vi "Actor Core.vi"(8 "error in":errorcluster, 11 "State in":refnum<class "Operator.lvclass">) -> (0 "error out":errorcluster, 3 "Actor out":refnum<class "Actor.lvclass">)   [LabVIEW 2014, in "Operator.lvlib" / "Operator.lvclass"]
doc: "(<B>Filename</B>: Actor Framework.lvlib:Actor.lvclass:Actor Core.vi)\n\nThis override invokes Entry.vi on the initial state, prior to calling the parent Actor Core. Adding this behavior to Actor Core (instead of an override of Pre Launch Init.vi) allows the initial state to launch a nested actor as part of its entry behavior.\n\nReceives messages to the actor, reacts to them, and initiates any error handling that may shut the actor down.\n\nDescendant classes may override this VI to append parallel tasks for the actor to complete while it handles messages. Overrides use the Call Parent Method node."
uses:
  Operator.lvclass
  <vilib>/ActorFramework/Actor/Actor.lvclass
  Operator Messages/Get Operator Joystick State Msg/Get Operator Joystick State Msg.lvclass
  Operator.lvclass/Operator.ctl
  Joystick/Joystick Class/Joystick.lvclass
  Robot Actor Framework/System Actor/System Actor Class/System Actor.lvclass
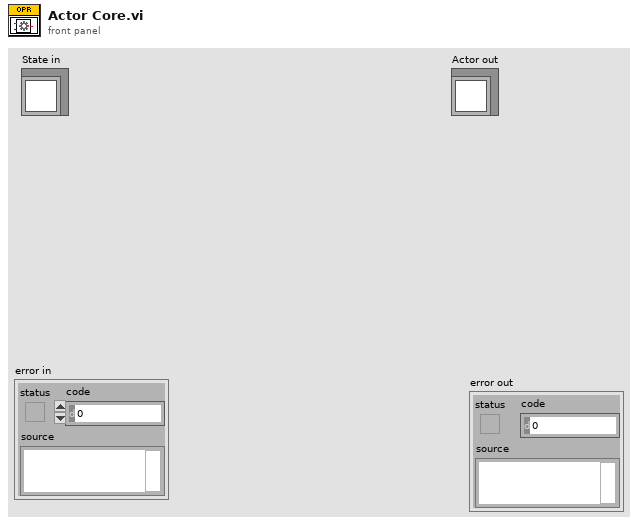
[diagram p1: front panel]
types:
  T1 = enum16{"Critical", "Error", "Warning", "Informational", "Debug"}
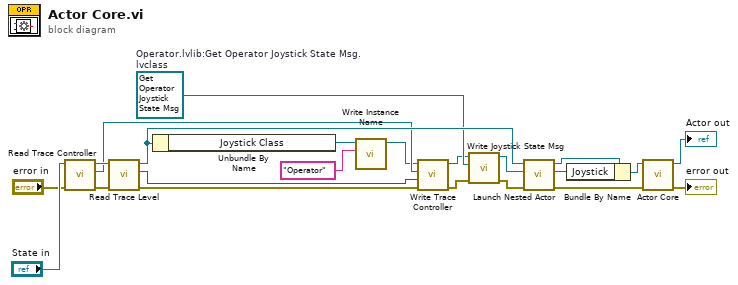
[diagram p0: block diagram]
diagram:
  w5 = refnum<class "Get Operator Joystick State Msg.lvclass"> refnum  # Operator.lvlib:Get Operator Joystick State Msg.lvclass
  n1 = call-dynamic "Read Trace Controller.vi"("error in (no error)"="error in", "System Actor in"="State in") -> ("error out"=w12:errorcluster, "Trace Controller"=w17:refnum<class "Message Enqueuer.lvclass">, "System Actor out"=w19:refnum<class "Operator.lvclass">)  [unwired: 7 in]
  n2 = call-dynamic "Read Trace Level.vi"("error in (no error)"=w12, "System Actor in"=w19) -> ("error out"=w11:errorcluster, "Trace Level"=w4:T1, "System Actor out"=w18:refnum<class "Operator.lvclass">)  [unwired: 7 in]
  n3 = Unbundle By Name(w18) -> ("Joystick Class"=w9:refnum<class "Joystick.lvclass">)
  n4 = call-dynamic "Write Instance Name.vi"("Instance Name"="Operator", "System Actor in"=w9) -> ("System Actor out"=w7:refnum<class "Joystick.lvclass">)  [unwired: 8 in, 1 out]
  n5 = call-dynamic "Write Trace Controller.vi"("error in (no error)"=w11, "Trace Level"=w4, "Trace Controller"=w17, "System Actor in"=w7) -> ("error out"=w2:errorcluster, "System Actor out"=w3:refnum<class "Joystick.lvclass">)  [unwired: 6 in]
  n6 = call-dynamic "Write Joystick State Msg.vi"("error in (no error)"=w2, "Joystick.lvlib:Get Joystick State Msg.lvclass"=w5, "Joystick in"=w3) -> ("error out"=w1:errorcluster, "Joystick out"=w6:refnum<class "Joystick.lvclass">)  [unwired: 7 in]
  n7 = call <vilib>:"Launch Nested Actor.vi"("error in (no error)"=w1, "Nested Actor"=w6, "Caller Actor in"=w18) -> ("error out"=w10:errorcluster, "Nested Actor's Enqueuer"=w15:refnum<class "Message Enqueuer.lvclass">, "Caller Actor out"=w14:refnum<class "Operator.lvclass">)  [unwired: 6 in]
  n8 = Bundle By Name(cluster=w14, "Joystick"=w15) -> (w16:refnum<class "Operator.lvclass">)
  n9 = call-parent "Actor Core.vi"("error in"=w10, "State in"=w16) -> ("error out"=→"error out":errorcluster, "Actor out"=→"Actor out":refnum<class "Actor.lvclass">)  [unwired: 8 in]
